vi "Run Test.vi"(8 "error in (no error)":errorcluster, 11 "CCT Test in":refnum<class "CTT Programming Test.lvclass">) -> (0 "error out":errorcluster, 1 "Fail Codes":string[](array[string]), 2 "Tests Passed":bool[](array[boolean]), 3 "CCT Test out":refnum<class "CTT Programming Test.lvclass">)   [LabVIEW 2015, in "CTT Programming Test.lvclass"]
uses:
  CTT Programming Test.lvclass
  Classes/Application/Class/Application.lvclass
  CT Common Tests/CT Common Tests.lvclass
  Test Class/Test Class.lvclass
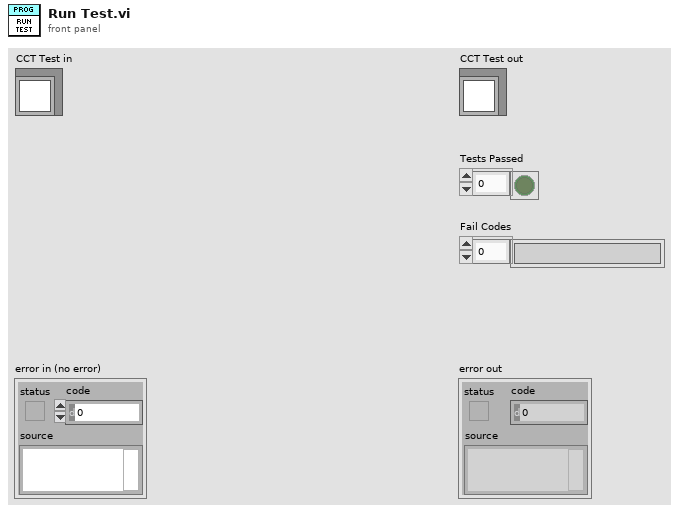
[diagram p1: front panel]
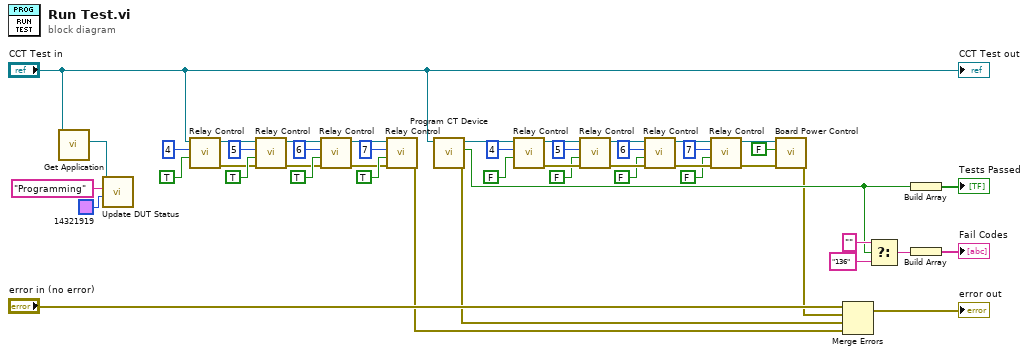
[diagram p0: block diagram]
diagram:
  n1 = call "Get Application.vi"("Test Class in"="CCT Test in") -> ("Application.lvlib:Application.lvclass"=w38:refnum<class "Application.lvclass">)  [unwired: 9 in, 1 out]
  n2 = call "Update DUT Status.vi"("BG Color"=u32 14321919, "Message ('')"="Programming", "Application in"=w38) -> ()  [unwired: 7 in, 2 out]
  n3 = call "Relay Control.vi"("State"=TRUE, "Channel (0)"=u32 4, "CT Common Tests in"="CCT Test in") -> ("error out"=w24:errorcluster, "CT Common Tests out"=w29:refnum<class "CTT Programming Test.lvclass">)  [unwired: 7 in]
  n4 = call "Relay Control.vi"("error in (no error)"=w24, "State"=TRUE, "Channel (0)"=u32 5, "CT Common Tests in"=w29) -> ("error out"=w25:errorcluster, "CT Common Tests out"=w28:refnum<class "CTT Programming Test.lvclass">)  [unwired: 6 in]
  n5 = call "Relay Control.vi"("error in (no error)"=w25, "State"=TRUE, "Channel (0)"=u32 6, "CT Common Tests in"=w28) -> ("error out"=w26:errorcluster, "CT Common Tests out"=w27:refnum<class "CTT Programming Test.lvclass">)  [unwired: 6 in]
  n6 = call "Relay Control.vi"("error in (no error)"=w26, "State"=TRUE, "Channel (0)"=u32 7, "CT Common Tests in"=w27) -> ("error out"=w2:errorcluster)  [unwired: 6 in, 1 out]
  n7 = call "Program CT Device.vi"("CTT Programming Test in"="CCT Test in") -> ("error out"=w1:errorcluster, "Passed"=w23:bool, "CTT Programming Test out"=w8:refnum<class "CTT Programming Test.lvclass">)  [unwired: 8 in]
  n8 = call "Relay Control.vi"("State"=FALSE, "Channel (0)"=u32 4, "CT Common Tests in"=w8) -> ("error out"=w22:errorcluster, "CT Common Tests out"=w17:refnum<class "CTT Programming Test.lvclass">)  [unwired: 7 in]
  n9 = call "Relay Control.vi"("error in (no error)"=w22, "State"=FALSE, "Channel (0)"=u32 5, "CT Common Tests in"=w17) -> ("error out"=w21:errorcluster, "CT Common Tests out"=w18:refnum<class "CTT Programming Test.lvclass">)  [unwired: 6 in]
  n10 = call "Relay Control.vi"("error in (no error)"=w21, "State"=FALSE, "Channel (0)"=u32 6, "CT Common Tests in"=w18) -> ("error out"=w20:errorcluster, "CT Common Tests out"=w19:refnum<class "CTT Programming Test.lvclass">)  [unwired: 6 in]
  n11 = call "Relay Control.vi"("error in (no error)"=w20, "State"=FALSE, "Channel (0)"=u32 7, "CT Common Tests in"=w19) -> ("error out"=w6:errorcluster, "CT Common Tests out"=w7:refnum<class "CTT Programming Test.lvclass">)  [unwired: 6 in]
  n12 = call "Board Power Control.vi"("error in (no error)"=w6, "Power-On"=FALSE, "CT Common Tests"=w7) -> ("error out"=w4:errorcluster)  [unwired: 7 in, 1 out]
  n13 = Merge Errors("error in (no error)", w4, w1, w2) -> (→"error out":errorcluster)
  n14 = Select(t="", s=w23, f="136") -> (s? t:f=w43:string)
  n15 = Build Array(w23) -> (→"Tests Passed":bool[])
  n16 = Build Array(w43) -> (→"Fail Codes":string[])
  "CCT Test out" <- "CCT Test in"
